vi "waveform.vi"() -> ()   [LabVIEW 2018]
uses:
  <vilib>/rvi/Emulation/niFpgaGetClockAttributes.vi
  <vilib>/rvi/Emulation/niFpgaSctlEmulationGetInTimedLoop.vi
  <vilib>/rvi/Emulation/niFpgaEmulationReportErrorSimple.vi
  <vilib>/rvi/Emulation/niFpgaCriticalErrorInLSC.vi
panel:
  in  "waveform_i64":i64[](array[numeric])=[0, 0, 0]
  out "waveform_i64":i64[](array[numeric])
  in  "waveform_i8":i8[](array[numeric])=[0, 0, 0]
  out "waveform_i8":i8[](array[numeric])
  in  "waveform_i32":i32[](array[numeric])=[0, 0, 0]
  out "waveform_i32":i32[](array[numeric])
  in  "waveform_i16":i16[](array[numeric])=[0, 0, 0]
  out "waveform_i16":i16[](array[numeric])
  in  "waveform_u8":u8[](array[numeric])=[0, 0, 0]
  out "waveform_u8":u8[](array[numeric])
  in  "waveform_u16":u16[](array[numeric])=[0, 0, 0]
  out "waveform_u16":u16[](array[numeric])
  in  "waveform_sgl":sgl[](array[numeric])=[0.0, 0.0, 0.0]
  in  "waveform_u64":u64[](array[numeric])=[0, 0, 0]
  out "waveform_sgl":sgl[](array[numeric]) format="%.2f"
  out "waveform_u64":u64[](array[numeric])
  out "waveform_u32":u32[](array[numeric])
  in  "waveform_u32":u32[](array[numeric])=[0, 0, 0]
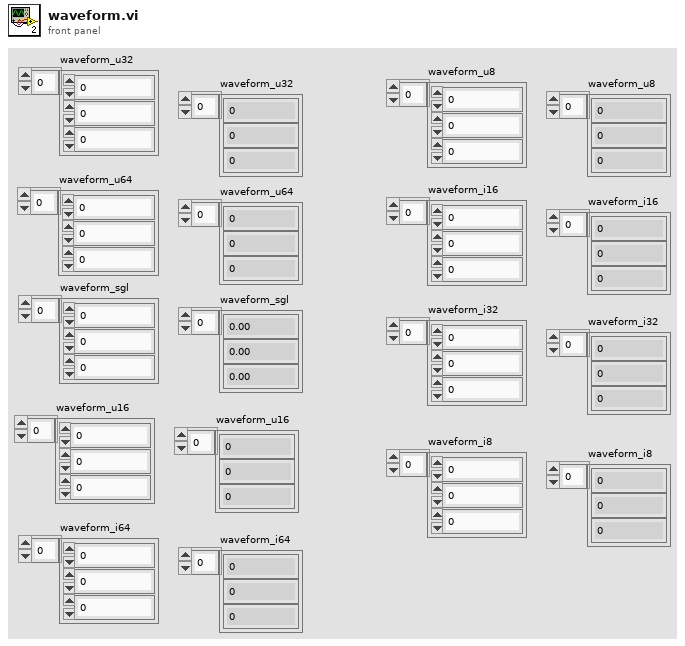
[diagram p1: front panel]
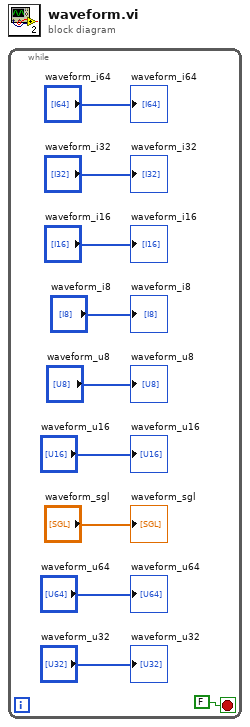
[diagram p0: block diagram]
diagram:
  n1 = while {
    stop <- FALSE stop-if-true
    "waveform_u32" <- "waveform_u32"
    "waveform_u64" <- "waveform_u64"
    "waveform_sgl" <- "waveform_sgl"
    "waveform_u16" <- "waveform_u16"
    "waveform_u8" <- "waveform_u8"
    "waveform_i8" <- "waveform_i8"
    "waveform_i16" <- "waveform_i16"
    "waveform_i32" <- "waveform_i32"
    "waveform_i64" <- "waveform_i64"
  }
